vi "SmartSEM Remote API initialization status.vi"(8 "error in":errorcluster, 11 "Api in":refnum<k7>(container)) -> (0 "error out":errorcluster, 1 "API initialized":bool, 3 "Api out":refnum<k7>)   [LabVIEW 2018]
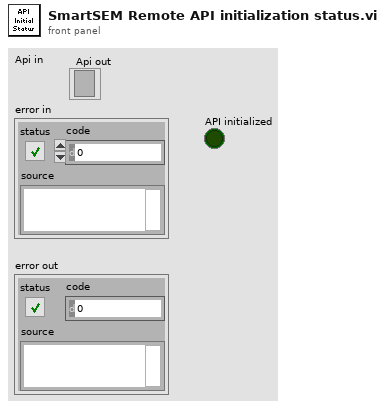
[diagram p1: front panel]
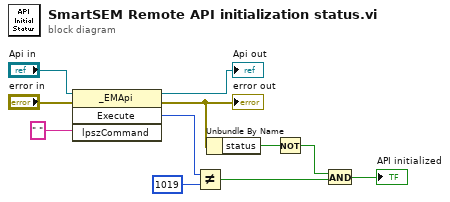
[diagram p0: block diagram]
diagram:
  n1 = invoke class="_EMApi" method="Execute"(reference="Api in", error in="error in", "lpszCommand"=" " ("lpszUserName")) -> (reference out=→"Api out":refnum<k7>, error out=w5:errorcluster, "Execute"=w10:i32)  [unwired: 1 in, 1 out]
  "error out" <- w5
  n2 = Not Equal?(x=w10, y=1019) -> (x != y?=w1:bool)
  n3 = Unbundle By Name(w5) -> ("status"=w4:bool)
  n4 = Not(x=w4) -> (.not. x?=w2:bool)
  n5 = And(x=w2, y=w1) -> (x .and. y?=→"API initialized":bool)
